vi "Polynomdaten auslesen PMA.vi"(8 "error in (no error)":errorcluster caption="Fehler (Eingang, kein Fehler)") -> (0 "error out":errorcluster caption="Fehler (Ausgang)", 1 "Aktiv":bool, 3 "Teil-Array":dbl[](array[numeric]))   [LabVIEW 2020, in "ABB-EL3000.lvlib" / "PMA.lvlib"]
uses:
  PMA.lvlib
  Analysator Definition/FGV Analysator Definition Aktionen.ctl
  Linearisierung V2/Aktionen Polynom Daten speichern.ctl
  FT-IR/FGV FT-IR Gasliste Aktionen.ctl
  Linearisierung V2/Linearisierung v2.lvlib
  Analysator Definition/Analysator Definition.lvlib
  Gaszuordnung AO/Gaszuordnung AO.lvlib
  FT-IR/FT-IR.lvlib
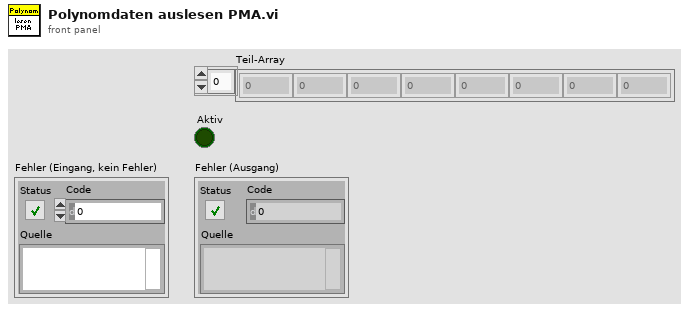
[diagram p1: front panel]
types:
  T1 = typedef "FT-IR.lvlib/FGV FT-IR Gasliste Aktionen.ctl" = enum16{"lesen", "Gasliste FT-IR", "Gasliste ausgelesen", "laden", "speichern", "löschen"}
  T2 = typedef "Linearisierung v2.lvlib/Aktionen Polynom Daten speichern.ctl" = enum16{"lesen", "laden", "speichern", "schreiben", "schreiben alle", "Liste erstellen", "aktivieren", "deaktivieren", "aktiv abfragen"}
  T3 = typedef "Analysator Definition.lvlib/FGV Analysator Definition Aktionen.ctl" = enum16{"lesen", "MB setzen", "MB KAL setzen", "laden"}
  T4 = typedef "Analysator Definition.lvlib/Betriebsdaten Komponente.ctl" = cluster{"Namen":string[], "MB Namen":string[], "Einheit":string, "MB Aktuell":u16, "MB Endwert":u16, "CalGase":u16[], "MB für KAL":u16[], "CG für KAL":u16[]}
  T5 = typedef "String - Ausgabefeld.ctl" = string
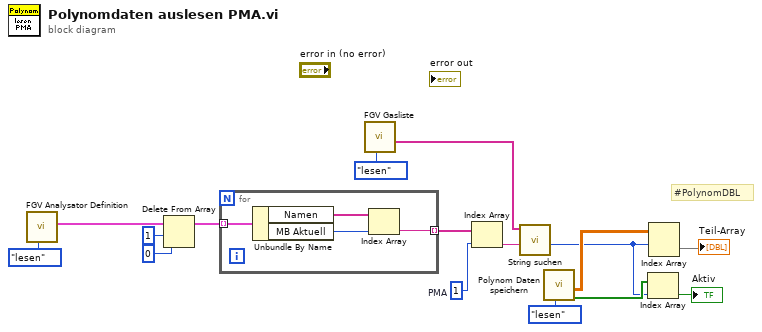
[diagram p0: block diagram]
diagram:
  w9 = 1  # PMA
  # "#PolynomDBL"
  n1 = call "FGV Analysator Definition.vi"("Aktionen"=FGV_Analysator_Definition_Aktionen."lesen") -> ("Betriebsdaten"=w13:T4[])  [unwired: 6 in, 4 out]
  n2 = Delete From Array(array=w13, length=1 ("Länge"), index=0 ("Index")) -> (array with subset deleted=w16:T4[])  [unwired: 1 out]
  n3 = for {
    tunnel: w16 -> [w20] mode=indexing
    tunnel: [w17] -> w10 mode=indexing
    n4 = Unbundle By Name(w20) -> ("Namen"=w19:string[], "MB Aktuell"=w18:u16)
    n5 = Index Array(array=w19, index=w18) -> (element=w17:string)
  }
  n6 = call "FGV Gasliste.vi"("Aktionen"=FGV_FT-IR_Gasliste_Aktionen."lesen") -> ("Aktuelle Gasliste gesamt"=w6:T5[])  [unwired: 8 in, 2 out]
  n7 = Index Array(array=w10, index=w9) -> (element=w8:string)
  n8 = call "String suchen.vi"("Gasname"=w8, "Such-Namen"=w6) -> ("Index"=w2:i32)  [unwired: 8 in, 1 out]
  n9 = call "Polynom Daten speichern.vi"("Aktionen"=Aktionen_Polynom_Daten_speichern."lesen") -> ("Aktiv"=w3:bool[], "Polynome"=w5:dbl[][])  [unwired: 5 in, 4 out]
  n10 = Index Array(array=w3, index=w2) -> (element=→"Aktiv":bool)
  n11 = Index Array(array=w5, index (row)=w2) -> (element=→"Teil-Array":dbl[])  [unwired: 1 in]
